vi "PictureRing.vi"() -> ()   [LabVIEW 2018]
panel:
  in  "Ring 2":u16(ring)
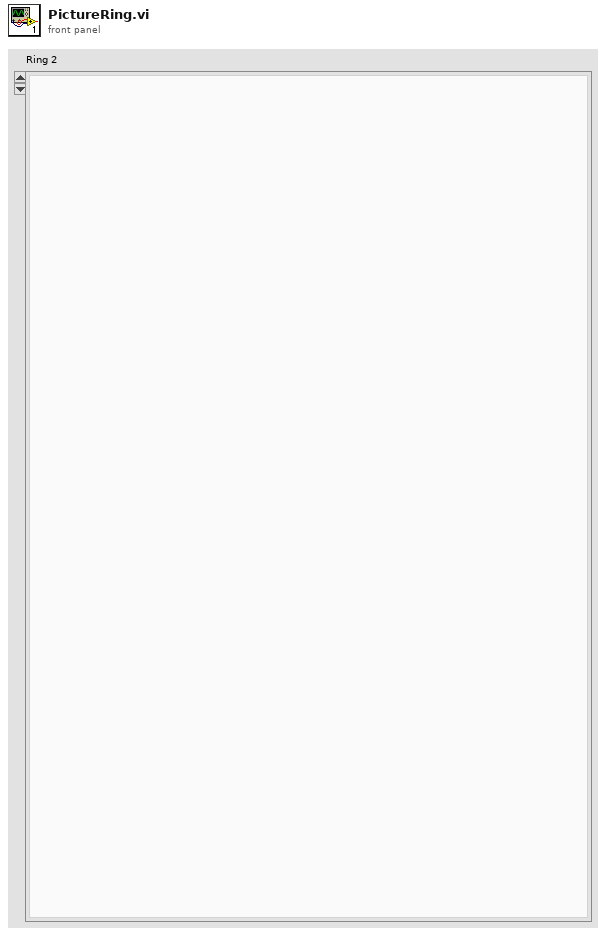
[diagram p1: front panel]
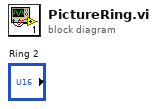
[diagram p0: block diagram]
diagram:
